vi "Filter Triggered.vi"(8 "error in (no error)":errorcluster, 10 "Assert Message":T1, 11 "Time Filters in":refnum<class "Time Filters.lvclass">) -> (0 "error out":errorcluster, 2 "Filtered":bool)   [LabVIEW 2018, in "Assert API Components.lvlib" / "Time Filters.lvclass"]
uses:
  Time Filters.lvclass
  Message Data.ctl
  Failure Actions.ctl
  Base Filter.lvclass
  Assert API Components.lvlib
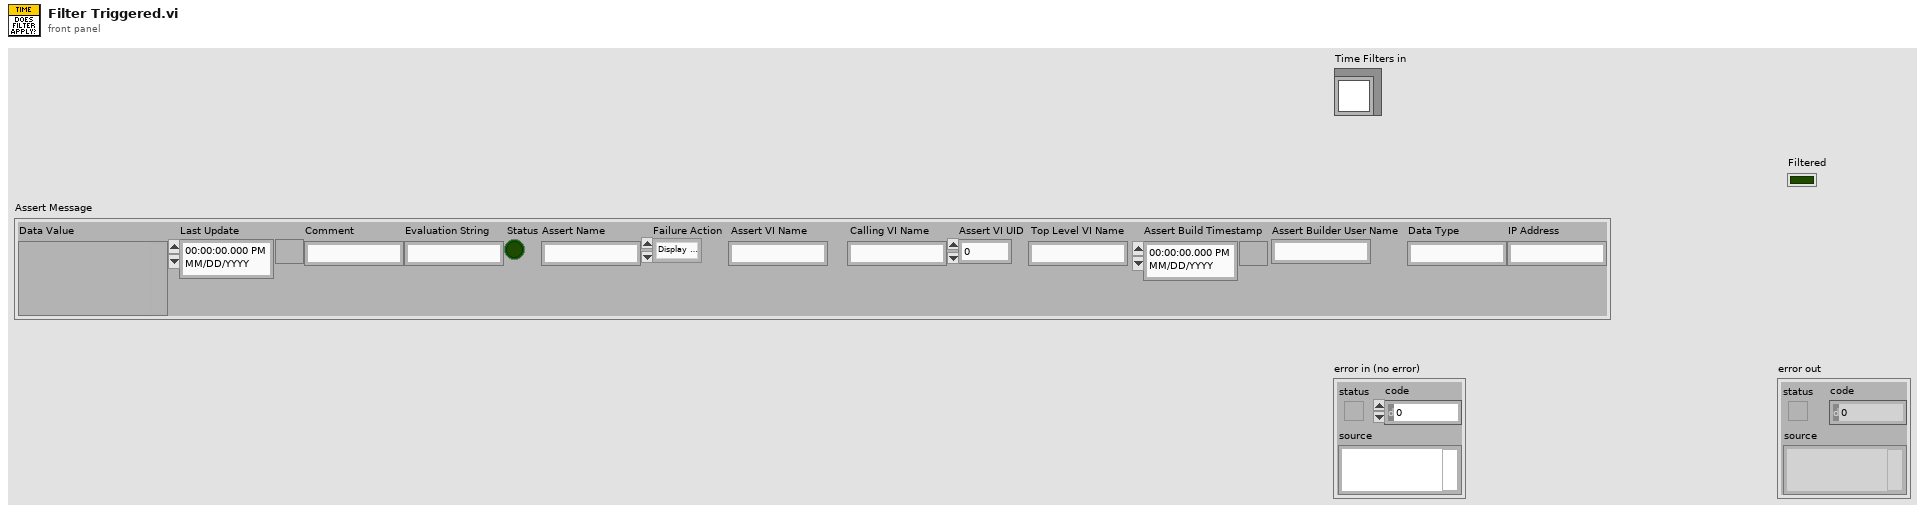
[diagram p1: front panel]
types:
  T1 = typedef "Assert API Components.lvlib/Message Data.ctl" = cluster{"Data Value":variant, "Last Update":timestamp, "Comment":string, "Evaluation String":string, "Status":bool, "Assert Name":string, "Failure Action":T2, "Assert VI Name":string, "Calling VI Name":string, "Assert VI UID":i32, "Top Level VI Name":string, "Assert Build Timestamp":timestamp, "Assert Builder User Name":string, "Data Type":string, "IP Address":string}
  T2 = typedef "Assert API Components.lvlib/Failure Actions.ctl" = enum16{"Display Only", "Log To File", "Pause Execution", "Abort Execution"}
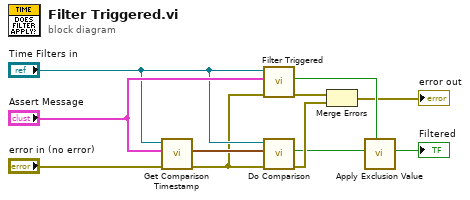
[diagram p0: block diagram]
diagram:
  n1 = call-dynamic "Get Comparison Timestamp.vi"("error in (no error)"="error in (no error)", "Assert Message"="Assert Message", "Time Filters in"="Time Filters in") -> ("error out"=w5:errorcluster, "Comparison Timestamp"=w6:timestamp)  [unwired: 7 in]
  n2 = call-parent "Filter Triggered.vi"("error in (no error)"=w5, "Assert Message"="Assert Message", "Base Filter in"="Time Filters in") -> ("error out"=w11:errorcluster, "Filtered"=w10:bool)  [unwired: 7 in]
  n3 = call "Do Comparison.vi"("error in (no error)"=w5, "Compare Timestamp"=w6, "Time Filters in"="Time Filters in") -> ("error out"=w3:errorcluster, "Filtered"=w1:bool)  [unwired: 7 in]
  n4 = Merge Errors(w11, w3) -> (→"error out":errorcluster)
  n5 = call "Apply Exclusion Value.vi"("Excluded?"=w10, "Filtered value in"=w1) -> ("Final Filtered Value"=→"Filtered":bool)  [unwired: 9 in]
